vi "GV AsyncTrigger.vi"() -> ()   [LabVIEW 2017]
panel:
  out "AsyncTrigger":bool
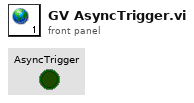
[diagram p1: front panel]
diagram:
